vi "PhotonPoseEstimator_Update.vi"(8 "Pass_Through_Time":dbl=-1.0 format="%33.4f", 11 "PhotonPoseEstimator":T10) -> (0 "New Data":bool, 1 "Pos Found":bool, 2 "PhotonEstimatedRobotPose":T1={"EstimatedPose"={"Translation3d"={"X"=0.0, "Y"=0.0, "Z"=0.0}, "Rotation3d"={"Q_quaternion"={"R"=1.0, "V"=[0.0, 0.0, 0.0]}}}, "TimeStamp_Seconds"=0.0, "targetsUsed"=[], "Strategy"=enum."LOWEST_AMBIGUITY"} {"targetsUsed"."AltCameraToTarget"."TRANSLATION3D"."Z" format="%14.3f"; "targetsUsed"."AltCameraToTarget"."TRANSLATION3D"."Y" format="%14.3f"; "targetsUsed"."AltCameraToTarget"."TRANSLATION3D"."X" format="%14.3f"; "targetsUsed"."BestCameraToTarget"."TRANSLATION3D"."Z" format="%14.3f"; "targetsUsed"."BestCameraToTarget"."TRANSLATION3D"."Y" format="%14.3f"; "targetsUsed"."BestCameraToTarget"."TRANSLATION3D"."X" format="%14.3f"; "EstimatedPose"."Translation3d"."Z" format="%14.3f"; "EstimatedPose"."Translation3d"."Y" format="%14.3f"; "EstimatedPose"."Translation3d"."X" format="%14.3f"}, 3 "out PhotonPoseEstimator":T10, 4 "Error Out":errorcluster)   [LabVIEW 2019, in "PhotonVisionLib.lvlib"]
doc: "Poll data from the configured cameras and update the estimated position of the robot. Returns empty if:\n - New data has not been received since the last call to {@code update()}.\n - No targets were found from the camera\n - There is no camera set\n\nInputs:\n -- PhotonPoseEstimator -- data cluster -- Data guiding how the position determination is done.\n -- PassThroughTime -- double -- FPGA time stamp in seconds. (Optional. Default: Read FPGA time.)\n\nOutputs:\n -- PhotonPoseEstimator -- data cluster -- Updated data cluster \n -- PhotonEstimatedRobotPose -- data cluster -- Estimated robot with an estimated pose, timestamp, and targets used to create the estimate.\n -- PosFound -- boolean -- A position has been determined.\n -- NewData -- boolean -- The data from photonvision is newer than the last time this routine was called."
uses:
  PhotonVisionLib.lvlib
  <vilib>/Rock Robotics/WPI/ThirdParty/JAS_Junk/TrajLib/TypeDef/TRANSLATION3D.ctl
  <vilib>/Rock Robotics/WPI/ThirdParty/JAS_Junk/TrajLib/Trajectory_Library.lvlib
  <vilib>/Rock Robotics/WPI/ThirdParty/JAS_Junk/TrajLib/TypeDef/QUATERNION.ctl
  <vilib>/Rock Robotics/WPI/ThirdParty/JAS_Junk/TrajLib/TypeDef/ROTATION3D.ctl
  <vilib>/Rock Robotics/WPI/ThirdParty/JAS_Junk/TrajLib/TypeDef/POSE3D.ctl
  TypeDef/PhotonEstimatedRobotPoseType.ctl
  Enum/PhotonPoseStrategy_ENUM.ctl
  TypeDef/TargetCornerType.ctl
  <vilib>/Rock Robotics/WPI/ThirdParty/JAS_Junk/TrajLib/TypeDef/TRANSFORM3D.ctl
  TypeDef/PhotonTrackedTargetType.ctl
  <vilib>/Rock Robotics/WPI/ThirdParty/JAS_Junk/TrajLib/TypeDef/AprilTag.ctl
  <vilib>/Rock Robotics/WPI/ThirdParty/JAS_Junk/TrajLib/Enum/AprilTagFieldLayoutOrignPosition_ENUM.ctl
  <vilib>/Rock Robotics/WPI/ThirdParty/JAS_Junk/TrajLib/TypeDef/AprilTagFieldLayout.ctl
  TypeDef/PhotonPoseEstimatorType.ctl
  TypeDef/PhotonTargetModel.ctl
  Ref/PhotonPoseEstimator_REF.ctl
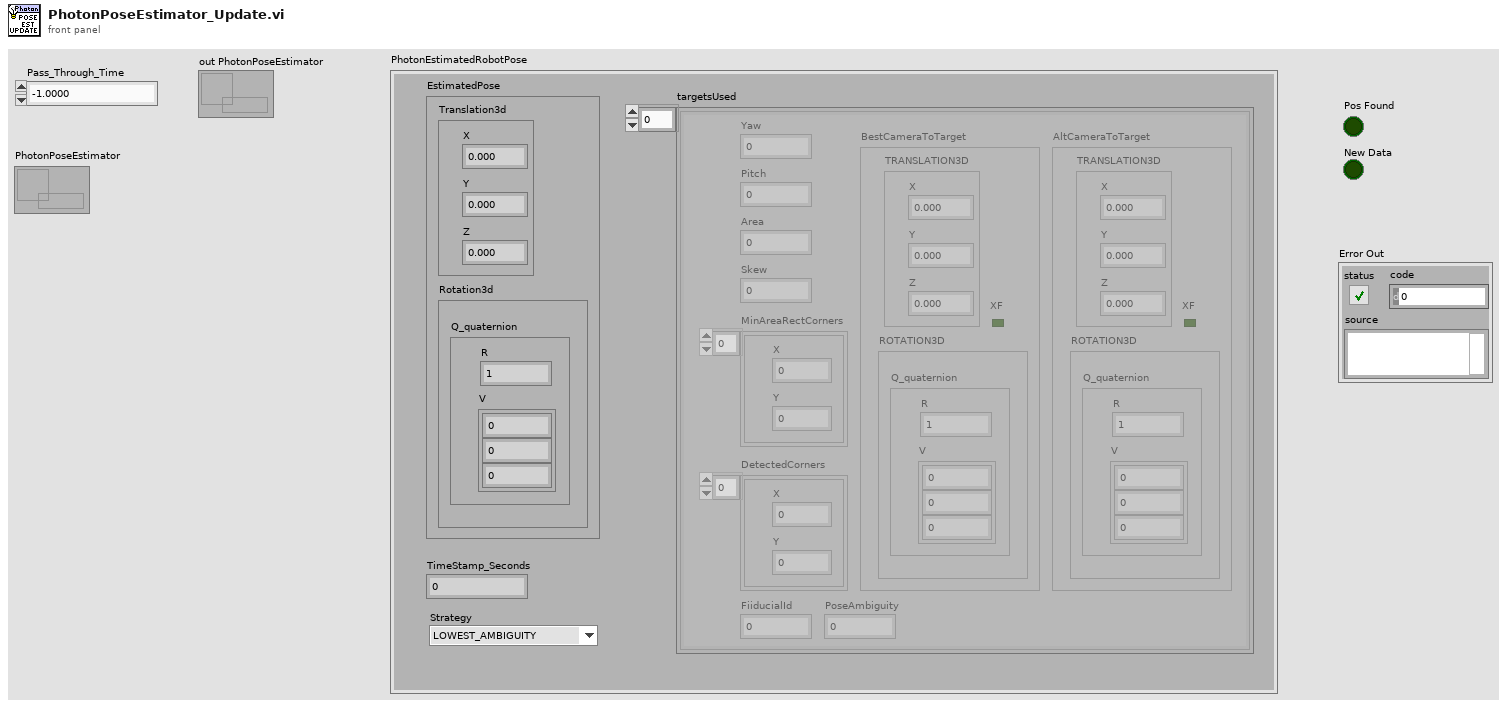
[diagram p1: front panel]
types:
  T1 = typedef "PhotonVisionLib.lvlib/PhotonEstimatedRobotPoseType.ctl" = cluster{"EstimatedPose":T2, "TimeStamp_Seconds":dbl, "targetsUsed":T6[], "Strategy":T9}
  T2 = typedef "Trajectory_Library.lvlib/POSE3D.ctl" = cluster{"Translation3d":T3, "Rotation3d":T4}
  T3 = typedef "Trajectory_Library.lvlib/TRANSLATION3D.ctl" = cluster{"X":dbl, "Y":dbl, "Z":dbl}
  T4 = typedef "Trajectory_Library.lvlib/ROTATION3D.ctl" = cluster{"Q_quaternion":T5}
  T5 = typedef "Trajectory_Library.lvlib/QUATERNION.ctl" = cluster{"R":dbl, "V":dbl[]}
  T6 = typedef "PhotonVisionLib.lvlib/PhotonTrackedTargetType.ctl" = cluster{"Yaw":dbl, "Pitch":dbl, "Area":dbl, "Skew":dbl, "MinAreaRectCorners":T7[], "BestCameraToTarget":T8, "FiiducialId":i32, "AltCameraToTarget":T8, "PoseAmbiguity":dbl, "DetectedCorners":T7[]}
  T7 = typedef "PhotonVisionLib.lvlib/TargetCornerType.ctl" = cluster{"X":dbl, "Y":dbl}
  T8 = typedef "Trajectory_Library.lvlib/TRANSFORM3D.ctl" = cluster{"TRANSLATION3D":T3, "ROTATION3D":T4, "XF":bool}
  T9 = typedef "PhotonVisionLib.lvlib/PhotonPoseStrategy_ENUM.ctl" = enum16{"LOWEST_AMBIGUITY", "CLOSEST_TO_CAMERA_HEIGHT", "CLOSEST_TO_REFERENCE_POSE", "CLOSEST_TO_LAST_POSE", "AVERAGE_BEST_TARGETS", "MULTI_TAG_PNP_ON_COPROCESSOR", "MULTI_TAG_PNP_ON_RIO"}
  T10 = typedef "PhotonVisionLib.lvlib/PhotonPoseEstimator_REF.ctl" = refnum<data-value>
  T11 = typedef "PhotonVisionLib.lvlib/PhotonPipelineResult_REF.ctl" = refnum<data-value>
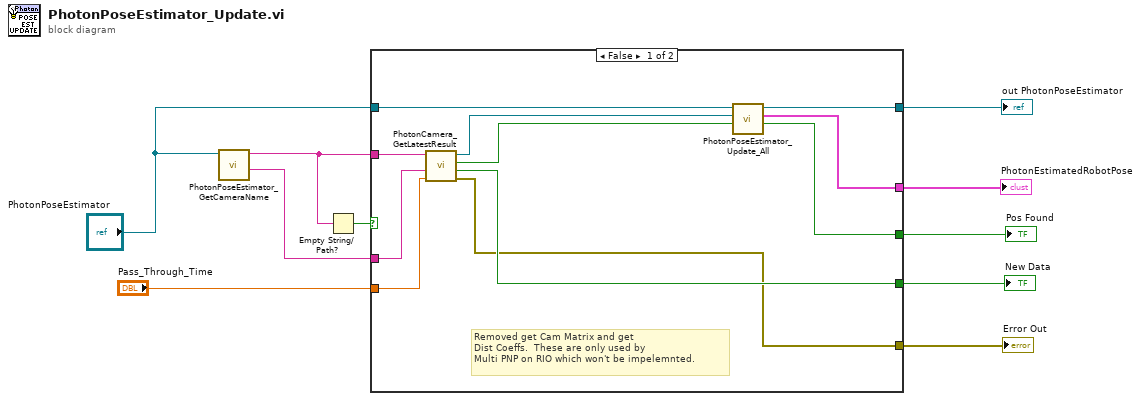
[diagram p0: block diagram]
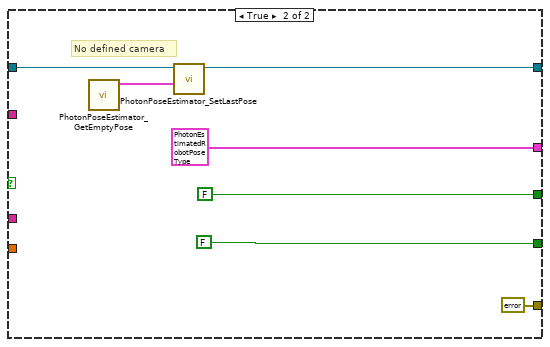
[diagram p2: hidden frame]
diagram:
  n1 = call "PhotonPoseEstimator_GetCameraName.vi"("PhotonPoseEstimator"="PhotonPoseEstimator") -> ("BaseNTName"=w1:string, "Camera"=w2:string)  [unwired: 9 in]
  n2 = Empty String/Path?(string/path=w2) -> (empty?=w10:bool)
  n3 = case shown="False" w10 {
    tunnel: "PhotonPoseEstimator" -> [w20 w24]
    tunnel: [w17 w23] -> w6
    tunnel: [w16 T1 {"EstimatedPose"={"Translation3d"={"X"=0.0, "Y"=0.0, "Z"=0.0}, "Rotation3d"={"Q_quaternion"={"R"=1.0, "V"=[0.0, 0.0, 0.0]}}}, "TimeStamp_Seconds"=0.0, "targetsUsed"=[], "Strategy"=enum."LOWEST_AMBIGUITY"} ("PhotonEstimatedRobotPose")] -> w7
    tunnel: w2 -> [w13 _]
    tunnel: [w15 FALSE] -> w9
    tunnel: [w21 FALSE ("New Data")] -> w8
    tunnel: "Pass_Through_Time" -> [w14 _]
    tunnel: [w11 errorcluster {"status"=FALSE, "code"=0, "source"=""} ("error IO")] -> w4
    tunnel: w1 -> [w12 _]
    frame False {
      # "Removed get Cam Matrix and get\nDist Coeffs.  These are only used by\nMulti PNP on RIO which won't be impelemnted."
      n4 = call "PhotonCamera_GetLatestResult.vi"("Pass_Through_Time"=w14, "BaseNTName"=w12, "CameraName"=w13) -> ("error out"=w11:errorcluster, "New Data"=w21:bool, "HasTargets"=w18:bool, "PipelineResult"=w19:T11)  [unwired: 5 in]
      n5 = call "PhotonPoseEstimator_Update_All.vi"("Has Results"=w18, "PipelineResult"=w19, "PhotonPoseEstimator"=w20) -> ("Pos Found"=w15:bool, "PhotonEstimatedRobotPose"=w16:T1, "out PhotonPoseEstimator"=w17:T10)  [unwired: 6 in]
    }
    frame True {
      # "No defined camera"
      n6 = call "PhotonPoseEstimator_GetEmptyPose.vi"() -> ("EmptyPose"=w25:T2)  [unwired: 11 in]
      n7 = call "PhotonPoseEstimator_SetLastPose.vi"("LastPose"=w25, "PhotonPoseEstimator"=w24) -> ("out PhotonPoseEstimator"=w23:T10)  [unwired: 9 in]
    }
  }
  "out PhotonPoseEstimator" <- w6
  "PhotonEstimatedRobotPose" <- w7
  "Pos Found" <- w9
  "New Data" <- w8
  "Error Out" <- w4
